vi "Day 9 Nested loops II.vi"() -> ()   [LabVIEW 2026]
panel:
  out "spreadsheet string 3":string
  in  "Pyramid Height (H)":i32
  out "concatenated string":string
  out "spreadsheet string 2":string
  out "spreadsheet string":string
  # "[H] Print a centred star pyramid (with leading spaces) of configurable \nheight."
  # "M] Reproduce the star triangle that grows 1 to 5 then shrinks 5 to 1, using \nnested loops / Case logic."
  # "[E] Print a left-aligned star triangle of height 5."
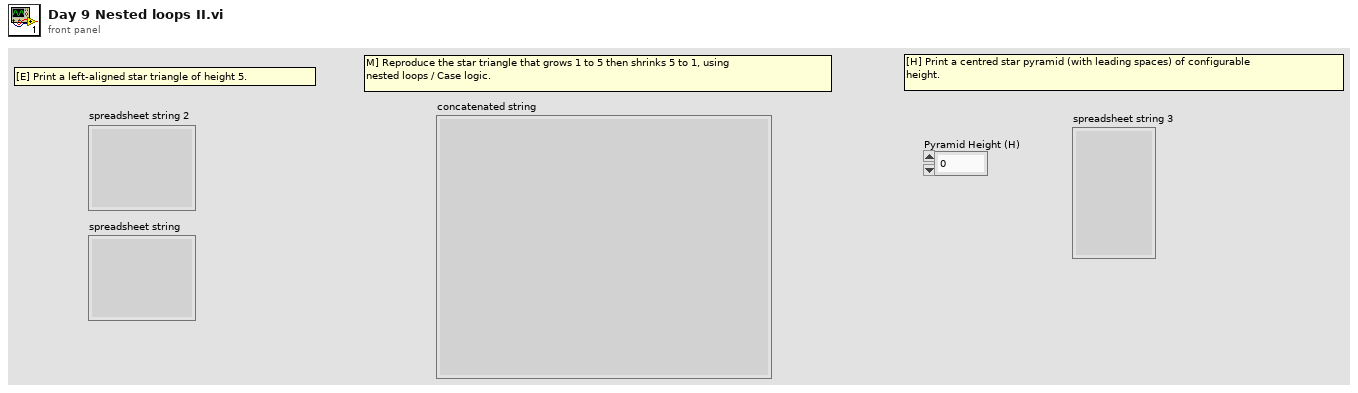
[diagram p1: front panel]
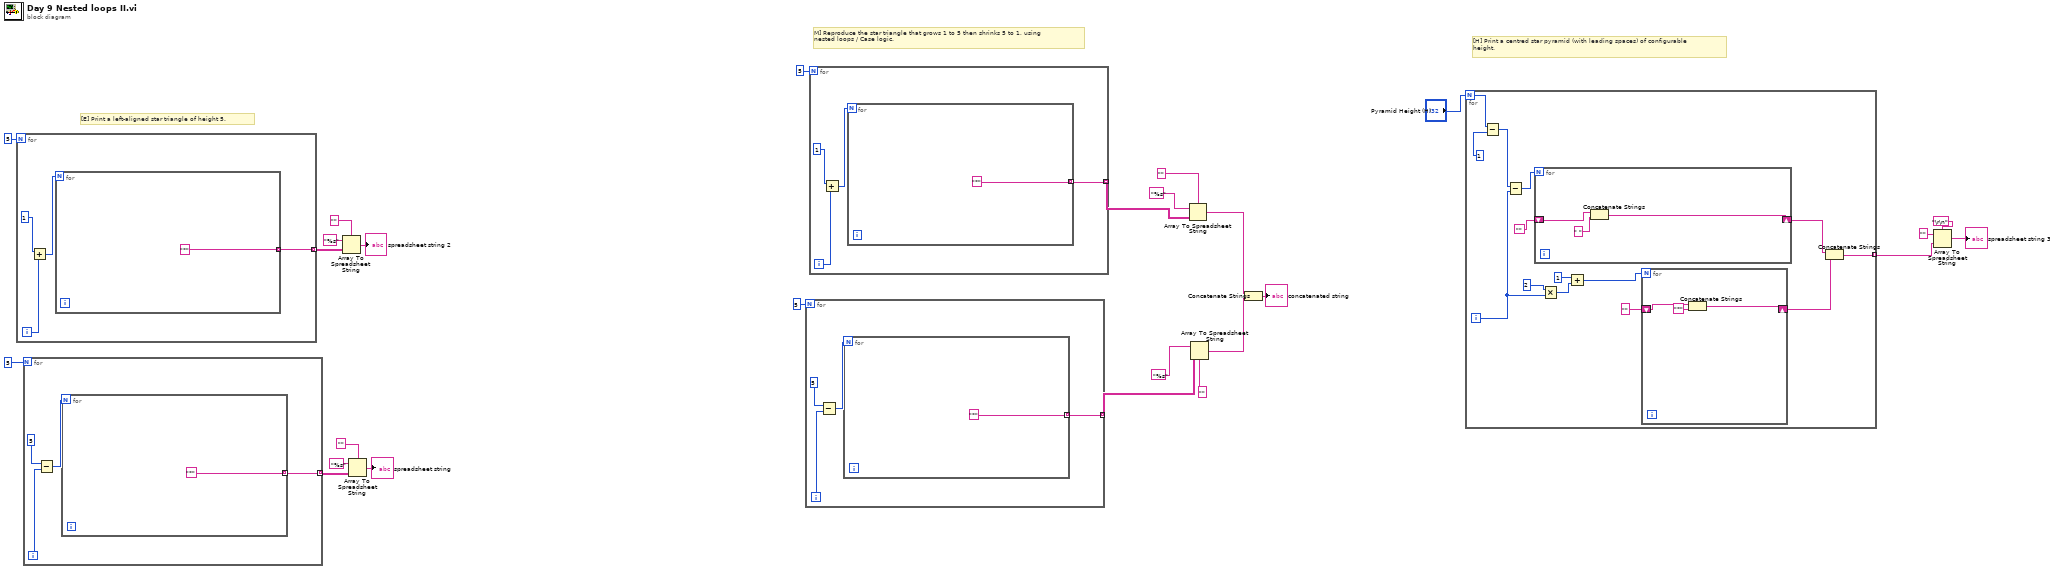
[diagram p0: block diagram]
diagram:
  # "[H] Print a centred star pyramid (with leading spaces) of configurable \nheight."
  # "M] Reproduce the star triangle that grows 1 to 5 then shrinks 5 to 1, using \nnested loops / Case logic."
  # "[E] Print a left-aligned star triangle of height 5."
  n1 = for {
    N: 5 -> [_]
    tunnel: [w30] -> w20 mode=indexing
    i -> [w29]
    n2 = Add(x=1, y=w29) -> (x+y=w27:i32)
    n3 = for {
      N: w27 -> [_]
      tunnel: ["*" ("String")] -> w30 mode=indexing
    }
  }
  n4 = for {
    N: 5 -> [_]
    tunnel: [w32] -> w25 mode=indexing
    i -> [w33]
    n5 = Subtract(x=5, y=w33) -> (x-y=w34:i32)
    n6 = for {
      N: w34 -> [_]
      tunnel: ["*" ("String")] -> w32 mode=indexing
    }
  }
  n7 = Array To Spreadsheet String(delimiter (Tab)="", array=w20, 3:"%s" ("format string")) -> (spreadsheet string=→"spreadsheet string 2":string)
  n8 = Array To Spreadsheet String(delimiter (Tab)="", array=w25, 3:"%s" ("format string")) -> (spreadsheet string=→"spreadsheet string":string)
  n9 = for {
    N: 5 -> [_]
    tunnel: [w37] -> w6 mode=indexing
    i -> [w38]
    n10 = Subtract(x=5, y=w38) -> (x-y=w39:i32)
    n11 = for {
      N: w39 -> [_]
      tunnel: ["*" ("String")] -> w37 mode=indexing
    }
  }
  n12 = for {
    N: 5 -> [_]
    tunnel: [w45] -> w7 mode=indexing
    i -> [w44]
    n13 = Add(x=1, y=w44) -> (x+y=w42:i32)
    n14 = for {
      N: w42 -> [_]
      tunnel: ["*" ("String")] -> w45 mode=indexing
    }
  }
  n15 = Array To Spreadsheet String(delimiter (Tab)="", array=w7, 3:"%s" ("format string")) -> (spreadsheet string=w10:string)
  n16 = Array To Spreadsheet String(delimiter (Tab)="", array=w6, 3:"%s" ("format string")) -> (spreadsheet string=w9:string)
  n17 = Concatenate Strings(w10, w9) -> (→"concatenated string":string)
  n18 = for {
    N: "Pyramid Height (H)" -> [w60]
    tunnel: [w47] -> w4 mode=indexing
    i -> [w55]
    n19 = Subtract(x=w60, y=1) -> (x-y=w58:i32)
    n20 = Subtract(x=w58, y=w55) -> (x-y=w57:i32)
    n21 = for {
      N: w57 -> [_]
      shift-right: [w64] -> w49
      shift-left: "" -> [w66]
      n22 = Concatenate Strings(w66, " ") -> (w64:string)
    }
    n23 = Multiply(x=2, y=w55) -> (x*y=w53:i32)
    n24 = Add(x=1, y=w53) -> (x+y=w51:i32)
    n25 = for {
      N: w51 -> [_]
      shift-right: [w61] -> w48
      shift-left: "" -> [w63]
      n26 = Concatenate Strings(w63, "*" ("string")) -> (w61:string)
    }
    n27 = Concatenate Strings(w49, w48) -> (w47:string)
  }
  n28 = Array To Spreadsheet String(delimiter (Tab)="\r\n", array=w4, 3:"" ("format string")) -> (spreadsheet string=→"spreadsheet string 3":string)
